vi "Open.vi"(8 "error in (no error)":errorcluster, 11 "MelsecTCP in":refnum<class "ModbusRtu.lvclass">) -> (0 "error out":errorcluster, 3 "MelsecTCP out":refnum<class "ModbusRtu.lvclass">)   [LabVIEW 2020, in "HslCommunication.lvlib" / "ModbusRtu.lvclass"]
uses:
  ModbusRtu.lvclass
  D:/Git/Labview-Libraries/Libraries/HslCommunication/Abstract PLC Controler/Abstract PLC Controler.lvclass
  EventLogger.lvlibp/1abvi3w/vi.lib/gpm_packages/@cs/event-logger/Source/Composed Log/Types/Log Level.ctl
  ModbusRtu.lvclass/ModbusRtu.ctl
  Abstract PLC Controler/Abstract PLC Controler.lvclass/Abstract PLC Controler.ctl
  D:/Git/Labview-Libraries/Libraries/HslCommunication/_Dependenciecs/HslCommunication.dll
  _Dependenciecs/HslCommunication.dll
  Abstract PLC Controler/Abstract PLC Controler.lvclass
  EventLogger.lvlibp/Logger.lvclass
  EventLogger.lvlibp/1abvi3w/vi.lib/gpm_packages/@cs/event-logger/Source/Composed Log/Composed Log.lvlib
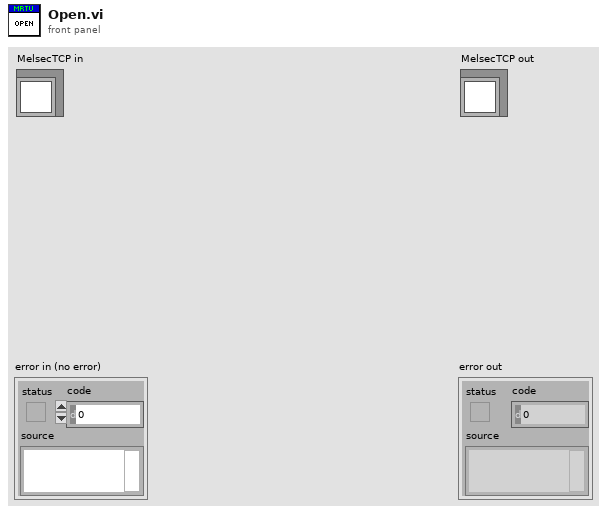
[diagram p1: front panel]
types:
  T1 = typedef "EventLogger.lvlibp/Composed Log.lvlib/Log Level.ctl" = enum16{"Debug", "Info", "Warning", "Error", "Critical"}
  T2 = cluster{"portName":string, "baudRate":i32, "dataBits":i32, "stopBits":i32, "parity":i32}
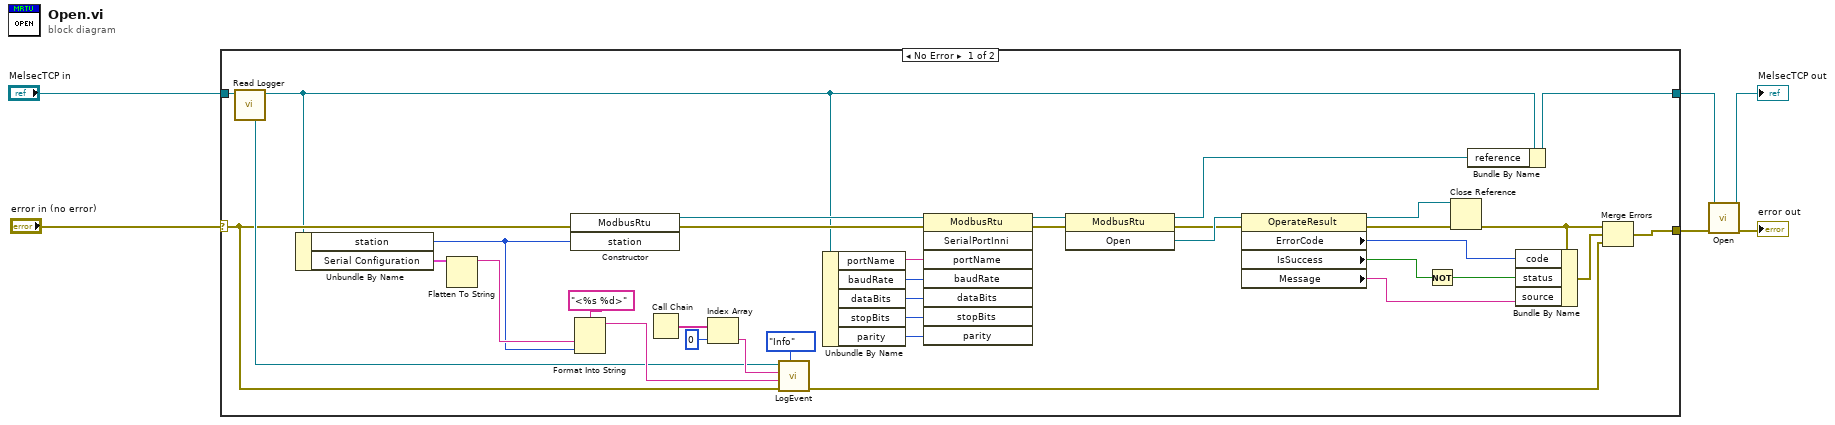
[diagram p0: block diagram]
diagram:
  n1 = case shown="No Error" "error in (no error)" {
    selector: "error in (no error)" -> [w22 w44]
    tunnel: "MelsecTCP in" -> [w42 w43]
    tunnel: [w41 w43] -> w2
    tunnel: [w35 w44] -> w4
    frame No Error {
      n2 = call "Read Logger.vi"("Abstract PLC Controler in"=w42) -> ("EventLogger.lvlibp:Logger.lvclass"=w23:refnum<class "Logger.lvclass">, "Abstract PLC Controler out"=w15:refnum<class "ModbusRtu.lvclass">)  [unwired: 9 in]
      n3 = Unbundle By Name(w15) -> ("station"=w7:u8, "Serial Configuration"=w9:T2)
      n4 = Flatten To String(anything=w9) -> (data string=w8:string)  [unwired: 3 in, 2 out]
      n5 = constructor class="ModbusRtu"(error in=w22, "station"=w7) -> (reference out=w32:refnum<k24>, error out=w31:errorcluster)  [unwired: 2 in, 2 out]
      n6 = Format Into String(format string="<%s %d>", w8, w7) -> (resulting string=w25:string)  [unwired: 2 in, 1 out]
      n7 = Call Chain() -> (call chain=w28:string[])
      n8 = Index Array(array=w28, index=0) -> (element=w24:string)
      n9 = call "LogEvent.vi"("Event Level"=Log_Level."Info", "error in (no error)"=w22, "Data To Log"=w25, "SourceID"=w24, "Logger in"=w23) -> ("error out"=w21:errorcluster)  [unwired: 5 in, 1 out]
      n10 = Unbundle By Name(w15) -> ("portName"=w10:string, "baudRate"=w14:i32, "dataBits"=w13:i32, "stopBits"=w12:i32, "parity"=w11:i32)
      n11 = invoke class="ModbusRtu" method="SerialPortInni"(reference=w32, error in=w31, "portName"=w10, "baudRate"=w14, "dataBits"=w13, "stopBits"=w12, "parity"=w11) -> (reference out=w29:refnum<k24>, error out=w18:errorcluster)  [unwired: 1 in, 6 out]
      n12 = invoke class="ModbusRtu" method="Open"(reference=w29, error in=w18) -> (reference out=w19:refnum<k24>, error out=w16:errorcluster, "Open"=w17:refnum<k24>)  [unwired: 1 in]
      n13 = property class="OperateResult"(reference=w17, error in=w16) -> (reference out=w34:refnum<k24>, error out=w33:errorcluster, "ErrorCode"=w38:i32, "IsSuccess"=w30:bool, "Message"=w36:string)
      n14 = Not(x=w30) -> (.not. x?=w37:bool)
      n15 = Close Reference(reference=w34, error in (no error)=w33) -> (error out=w39:errorcluster)
      n16 = Bundle By Name(cluster=w15, "reference"=w19) -> (w41:refnum<class "ModbusRtu.lvclass">)
      n17 = Bundle By Name(cluster=w39, "code"=w38, "status"=w37, "source"=w36) -> (w40:errorcluster)
      n18 = Merge Errors(w39, w40, w21) -> (w35:errorcluster)
    }
    frame Error {
    }
  }
  n19 = call-parent "Open.vi"("error in (no error)"=w4, "MelsecTCP in"=w2) -> ("error out"=→"error out":errorcluster, "MelsecTCP out"=→"MelsecTCP out":refnum<class "ModbusRtu.lvclass">)  [unwired: 8 in]
